vi "运维调试_总磷总氮.vi"() -> ()   [LabVIEW 2016, in "斯坦道仪器.lvlib"]
uses:
  <vilib>/Platform/TimedLoop/XDataNode/timing_clust.ctl
  <vilib>/Platform/TimedLoop/XDataNode/nitl_modes.ctl
  <vilib>/Platform/TimedLoop/XDataNode/wakeup.ctl
  <vilib>/Utility/miscctls.llb/LVPointTypeDef.ctl
  <vilib>/Utility/config.llb/Read Key (Double).vi
  <vilib>/Utility/config.llb/Write Key (Double).vi
  <vilib>/Platform/TimedLoop/XDataNode/XDataNode.xnode
  <vilib>/Platform/TimedLoop/XDataNode/XDNodeRunTimeDep.lvlib
  <vilib>/Utility/config.llb/NI_LVConfig.lvlib
panel:
  out "温度2":sgl
  out "温度1":sgl
  out "ADC":sgl
  out "字符串":string
  out "总氮稀释倍数":dbl
  out "固件版本号":string
  in  "数组":string[](array[string])
  in  "备用系数写入":bool
  in  "备用系数读取":bool
  in  "备用系数":T1
  in  "量程切换阈值写入":bool
  in  "量程切换阈值读取":bool
  in  "量程切换阈值":cluster{"阈值":dbl, "标液浓度":dbl}
  in  "参数下拉列表":enum16{"总磷", "总氮"}(ring)
  in  "量程下拉列表":enum16{"低量程", "高量程"}(ring)
  in  "测量模式下拉列表":enum16{"水样测量", "空白核查", "跨度核查", "标样核查", "加标回收"}(ring)
  in  "公式":cluster{"X^2":dbl, "X":dbl, "b":dbl}
  in  "写公式":bool
  in  "读公式":bool
  in  "精度":dbl=4.0
  in  "样品5 F0":dbl
  in  "样品5 F1":dbl
  in  "样品4 F1":dbl
  in  "样品4 F0":dbl
  in  "样品3 F0":dbl
  in  "样品3 F1":dbl
  in  "样品2 F0":dbl
  in  "样品2 F1":dbl
  in  "样品1 F1":dbl
  in  "样品1 F0":dbl
  in  "method":u16(ring) items=["最小二乘", "最小绝对残差", "Bisquare"]
  in  "模型":enum32{"线性", "多项式"}(ring)
  out "r^2":dbl format="%.7g"
  out "拟合公式":string
  in  "样品2启用":bool
  in  "样品5启用":bool
  in  "样品4启用":bool
  in  "样品3启用":bool
  in  "样品1启用":bool
  in  "标液浓度5":dbl
  out "测量吸光度5":dbl
  in  "标液浓度4":dbl
  out "测量吸光度4":dbl
  in  "标液浓度3":dbl
  out "测量吸光度3":dbl
  in  "标液浓度2":dbl
  out "测量吸光度2":dbl
  out "测量吸光度1":dbl
  in  "标液浓度1":dbl
  out "XY图":cluster{"X Values":dbl[], "Y Values":dbl[]}[](graph)
  in  "返回":bool
  in  "设置":bool
  out "序列号":string="序列号"
  out "总氮测量数据":T2(xcontrol)
  out "总磷测量数据":T2(xcontrol)
  out "集成报警信息":string
  out "设置值":dbl
  out "定时启动":bool
  out "总磷总氮运行状态":T3(xcontrol)
  in  "停止":bool
  in  "手动启动":bool
  in  "单步测试":bool
  in  "总磷氨氮调试":u16[](xcontrol)
  out "F3":sgl format="%#.6f"
  out "F2":sgl format="%#.6f"
  out "F1":sgl format="%#.6f"
  out "F0":sgl format="%#.6f"
  out "多列列表框":i32(listbox)
  # "COM5"
  # "参数设置"
  # "标液浓度"
  # "F0"
  # "F1"
  # "吸光值显示"
  # "样品一"
  # "辅\n助\n计\n算\n区"
  # "样品二"
  # "样品三"
  # "样品四"
  # "样品五"
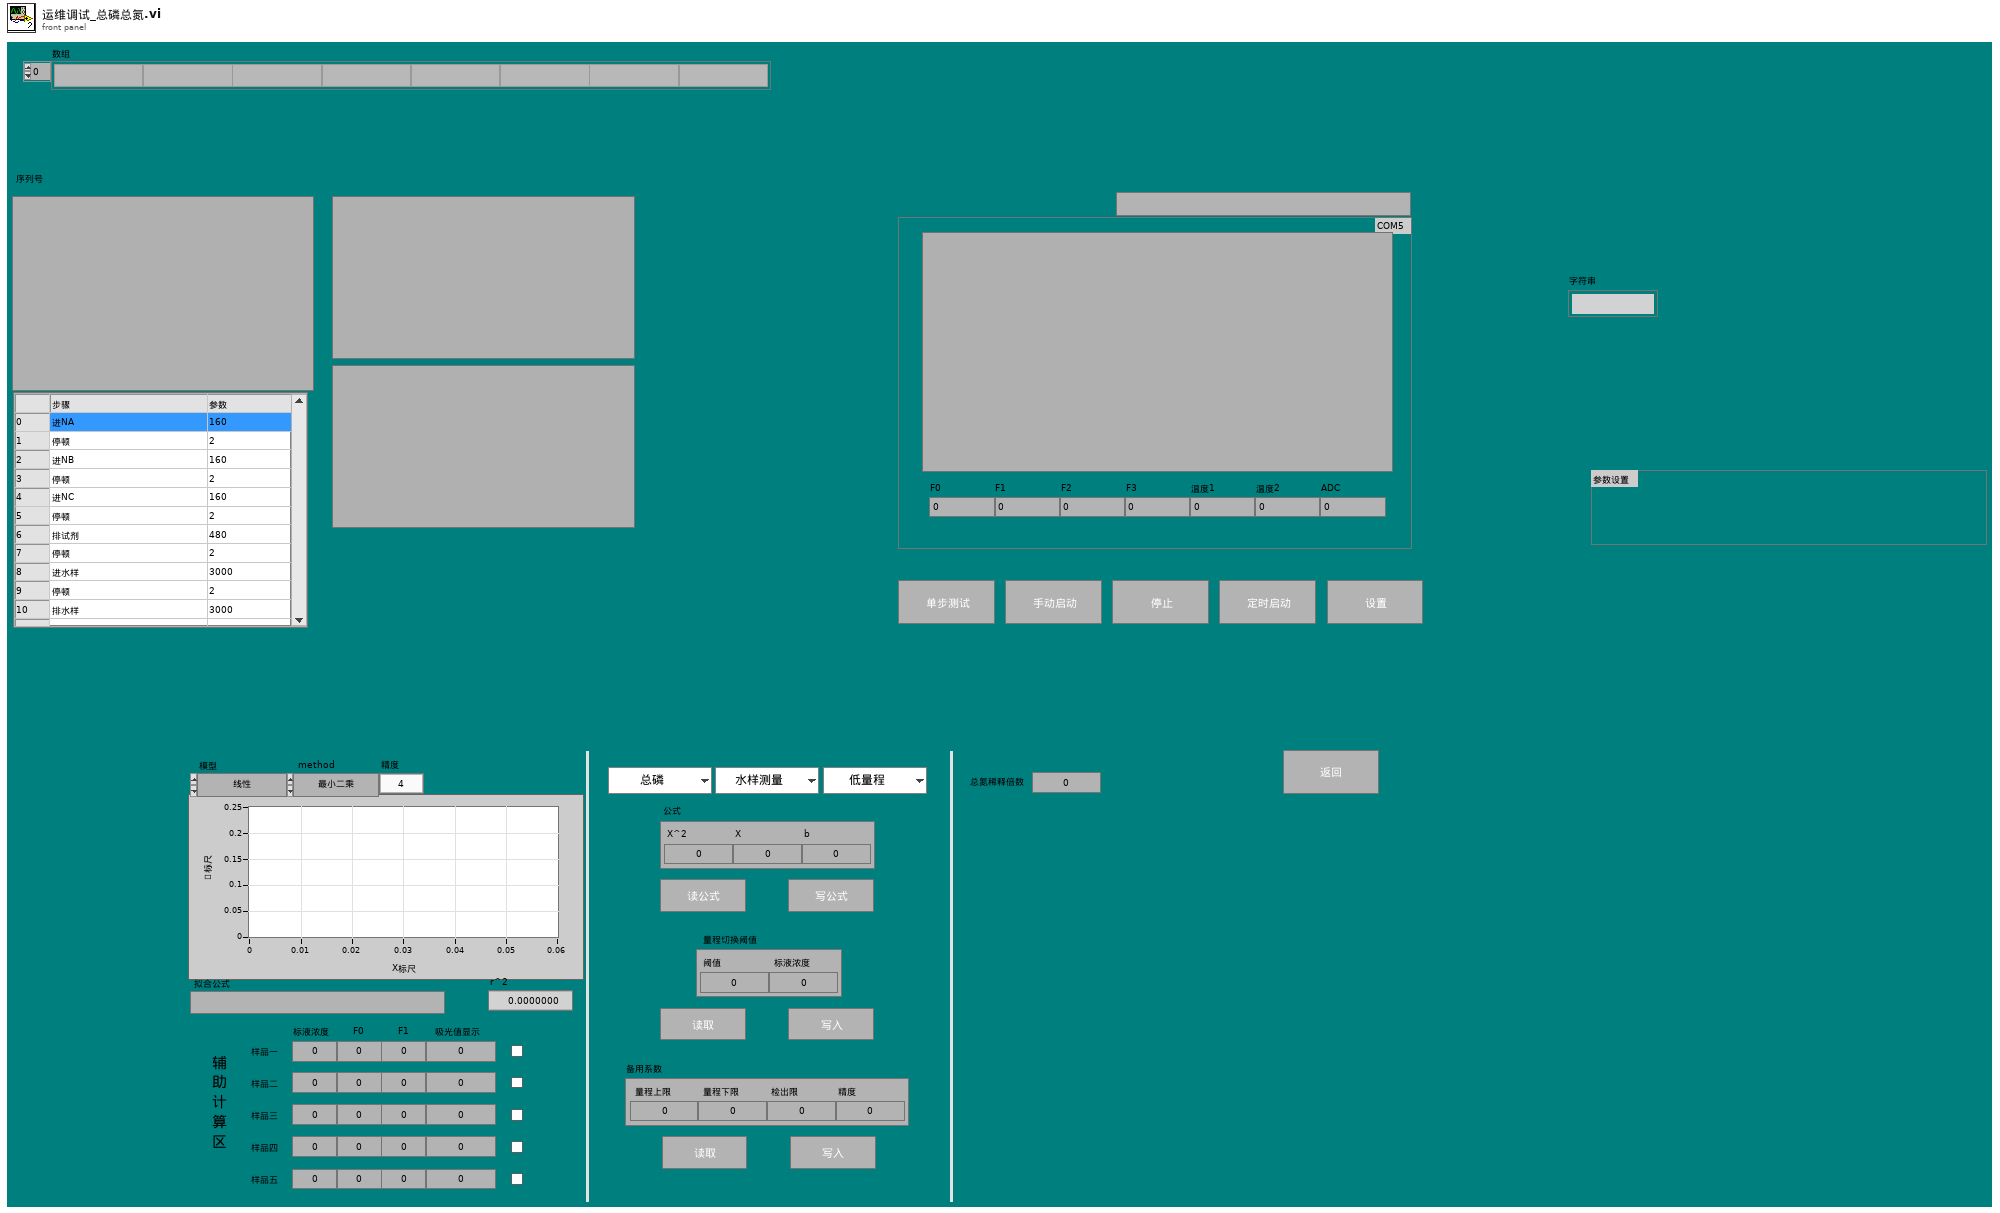
[diagram p1: front panel]
types:
  T1 = cluster{"量程上限":dbl, "量程下限":dbl, "检出限":dbl, "精度":dbl}
  T2 = cluster{"flowid":u16, "测量精度":u16, "测量数据区":cluster{"因子编码":u32, "单位":u16, "标样参考值":sgl, "水样数据时间":timestamp, "水样实测值":sgl, "水样数据标识":string, "标样数据时间":timestamp, "标样实测值":sgl, "标样数据标识":string, "空白数据时间":timestamp, "空白实测值":sgl, "空白数据标识":string, "零点核查数据时间":timestamp, "零点核查实测值":sgl, "零点核查数据标识":string, "跨度核查数据时间":timestamp, "跨度核查实测值":sgl, "跨度核查数据标识":string, "加标回收数据时间":timestamp, "加标回收实测值":sgl, "加标回收数据标识":string, "平行样数据时间":timestamp, "平行样实测值":sgl, "平行样数据标识":string, "F0":sgl, "F1":sgl, "F2":sgl, "F3":sgl, "F4":sgl, "F5":sgl, "F6":sgl, "F7":sgl, "温度":sgl, "湿度":sgl, "X值":sgl}}
  T3 = cluster{"系统时间":timestamp, "工作状态":enum16{"空闲", "水样测试", "标样核查", "零点核查", "跨度核查", "空白测试", "平行样测试", "加标回收", "空白校准", "标样校准", "初始化（清洗）"}, "测量模式":enum16{"待机", "连续模式", "周期模式", "定点模式", "受控模式", "手动模式"}, "告警代码":enum16{"无告警", "缺试剂告警", "缺水样告警", "缺蒸馏水告警", "缺标液告警", "仪表漏液告警", "标定异常告警", "超量程告警", "加热异常", "低试剂预警", "超上限告警", "超下限告警", "仪表内部其他异常", "滴定异常告警", "电极异常告警", "量程切换告警", "参数设置告警", "PH电极电位异常", "电导率电极异常", "浊度光度异常", "溶解氧电极异常", "溶解氧光强异常", "温度异常告警", "PH异常告警", "溶解氧异常告警", "电导率异常告警", "浊度异常告警", "叶绿素异常告警", "藻密度异常告警", "蓝绿藻异常告警", "ORP异常告警", "氨氮异常告警", "清洁刷异常告警", "SD卡异常告警", "蓝牙异常告警", "Wifi异常告警", "流程异常告警"}, "故障代码":enum16{"无故障", "电机故障", "温度故障", "通讯故障", "滴定故障"}, "日志代码":u16, "软件版本":u16, "F0":sgl, "F1":sgl, "F2":sgl, "F3":sgl, "T":sgl, "H":sgl, "id":u16, "flowid":u16, "量程":u16, "总磷控温温度1":sgl, "营养盐控温温度2":sgl, "ADC":sgl}
  T4 = enum16{"待机", "启动氨氮", "氨氮测量中", "启动总磷", "总磷测量中", "延时"}
  T5 = typedef "LVPointTypeDef.ctl" = cluster{"Horizontal":i16, "Vertical":i16}
  T6 = cluster{"因子编码":u32, "单位":u16, "标样参考值":sgl, "水样数据时间":timestamp, "水样实测值":sgl, "水样数据标识":string, "标样数据时间":timestamp, "标样实测值":sgl, "标样数据标识":string, "空白数据时间":timestamp, "空白实测值":sgl, "空白数据标识":string, "零点核查数据时间":timestamp, "零点核查实测值":sgl, "零点核查数据标识":string, "跨度核查数据时间":timestamp, "跨度核查实测值":sgl, "跨度核查数据标识":string, "加标回收数据时间":timestamp, "加标回收实测值":sgl, "加标回收数据标识":string, "平行样数据时间":timestamp, "平行样实测值":sgl, "平行样数据标识":string, "F0":sgl, "F1":sgl, "F2":sgl, "F3":sgl, "F4":sgl, "F5":sgl, "F6":sgl, "F7":sgl, "温度":sgl, "湿度":sgl, "X值":sgl}
  T7 = enum16{"空闲", "水样测试", "标样核查", "零点核查", "跨度核查", "空白测试", "平行样测试", "加标回收", "空白校准", "标样校准", "初始化（清洗）"}
  T8 = typedef "XDNodeRunTimeDep.lvlib/timing_clust.ctl" = cluster{"Expected End [f-1]":u64, "Actual End [f-1]":u64, "Finished Late? [f-1]":bool, "Expected End [i-1]":u64, "Actual End [i-1]":u64, "Finished Late? [i-1]":bool, "Expected Start [i]":u64, "Actual Start [i]":u64, "Expected Start [f]":u64, "Actual Start [f]":u64, "Source Name":string, "Structure Name":string, "Period":i64, "Deadline":i64, "Offset":i64, "Start":i64, "Priority":i32, "Timeout":i32, "Mode":T9, "Wakeup Reason":T10, "Error":errorcluster, "Source Type":string, "Secondary Source Type":string, "Global End Time":u64, "Global Start Time":u64, "Frame Duration":u64, "Iteration Duration":u64, "Assigned CPU":i32, "I/O Scan Engine Mode":u32}
  T9 = typedef "XDNodeRunTimeDep.lvlib/nitl_modes.ctl" = enum32{"No Change", "Process missed periods, maintain original phase", "Discard missed periods, maintain original phase", "Process missed periods, ignore original phase", "Discard missed periods, ignore original phase"}
  T10 = typedef "XDNodeRunTimeDep.lvlib/wakeup.ctl" = enum32{"Normal", "Aborted", "Asynchronous wakeup", "Timing source error", "Timed loop error", "Timeout"}
  T11 = cluster{"启动模式":enum16{"标液测量", "水样测量", "零液测量", "盲样测量", "加标回收"}, "启动参数":u16, "量程":enum16{"低量程", "高量程"}}
  T12 = cluster{"时间标识":timestamp, "设备":string, "日志信息":string, "流程参数":string}
  T13 = cluster{"时间标识":timestamp, "设备":string, "日志信息":string}
  T14 = enum16{"无告警", "缺试剂告警", "缺水样告警", "缺蒸馏水告警", "缺标液告警", "仪表漏液告警", "标定异常告警", "超量程告警", "加热异常", "低试剂预警", "超上限告警", "超下限告警", "仪表内部其他异常", "滴定异常告警", "电极异常告警", "量程切换告警", "参数设置告警", "PH电极电位异常", "电导率电极异常", "浊度光度异常", "溶解氧电极异常", "溶解氧光强异常", "温度异常告警", "PH异常告警", "溶解氧异常告警", "电导率异常告警", "浊度异常告警", "叶绿素异常告警", "藻密度异常告警", "蓝绿藻异常告警", "ORP异常告警", "氨氮异常告警", "清洁刷异常告警", "SD卡异常告警", "蓝牙异常告警", "Wifi异常告警", "流程异常告警"}
  T15 = typedef "LVRowAndColumnUnsignedTypeDef.ctl" = cluster{"Row":u32, "Column":u32}
  T16 = typedef "NI_LVConfig.lvlib/Config Data RefNum.ctl" = refnum<k1>
  T17 = cluster{"站号":u16, "量程切换":enum32{"H", "L", "AUTO"}, "控制命令":enum16{"启动测量", "标样核查", "零点核查", "跨度核查", "空白测试", "平行样测试", "加标回收", "空白校准", "标样校准", "初始化（清洗）", "停止测试", "仪器重启", "校时", "模式设置", "测量间隔设置"}, "模式设置":enum16{"待机", "连续模式", "周期模式", "定点模式", "受控模式", "手动模式"}, "测量间隔":u16}
  T18 = cluster{"站号":u16, "量程切换":enum32{"H", "L", "AUTO"}, "控制命令":enum16{"启动测量", "标样核查", "零点核查", "跨度核查", "空白测试", "平行样测试", "加标回收", "空白校准", "标样校准", "初始化（清洗）", "停止测试", "仪器重启", "校时", "模式设置", "测量间隔设置", "盲样测试"}, "模式设置":enum16{"待机", "连续模式", "周期模式", "定点模式", "受控模式", "手动模式"}, "测量间隔":u16}
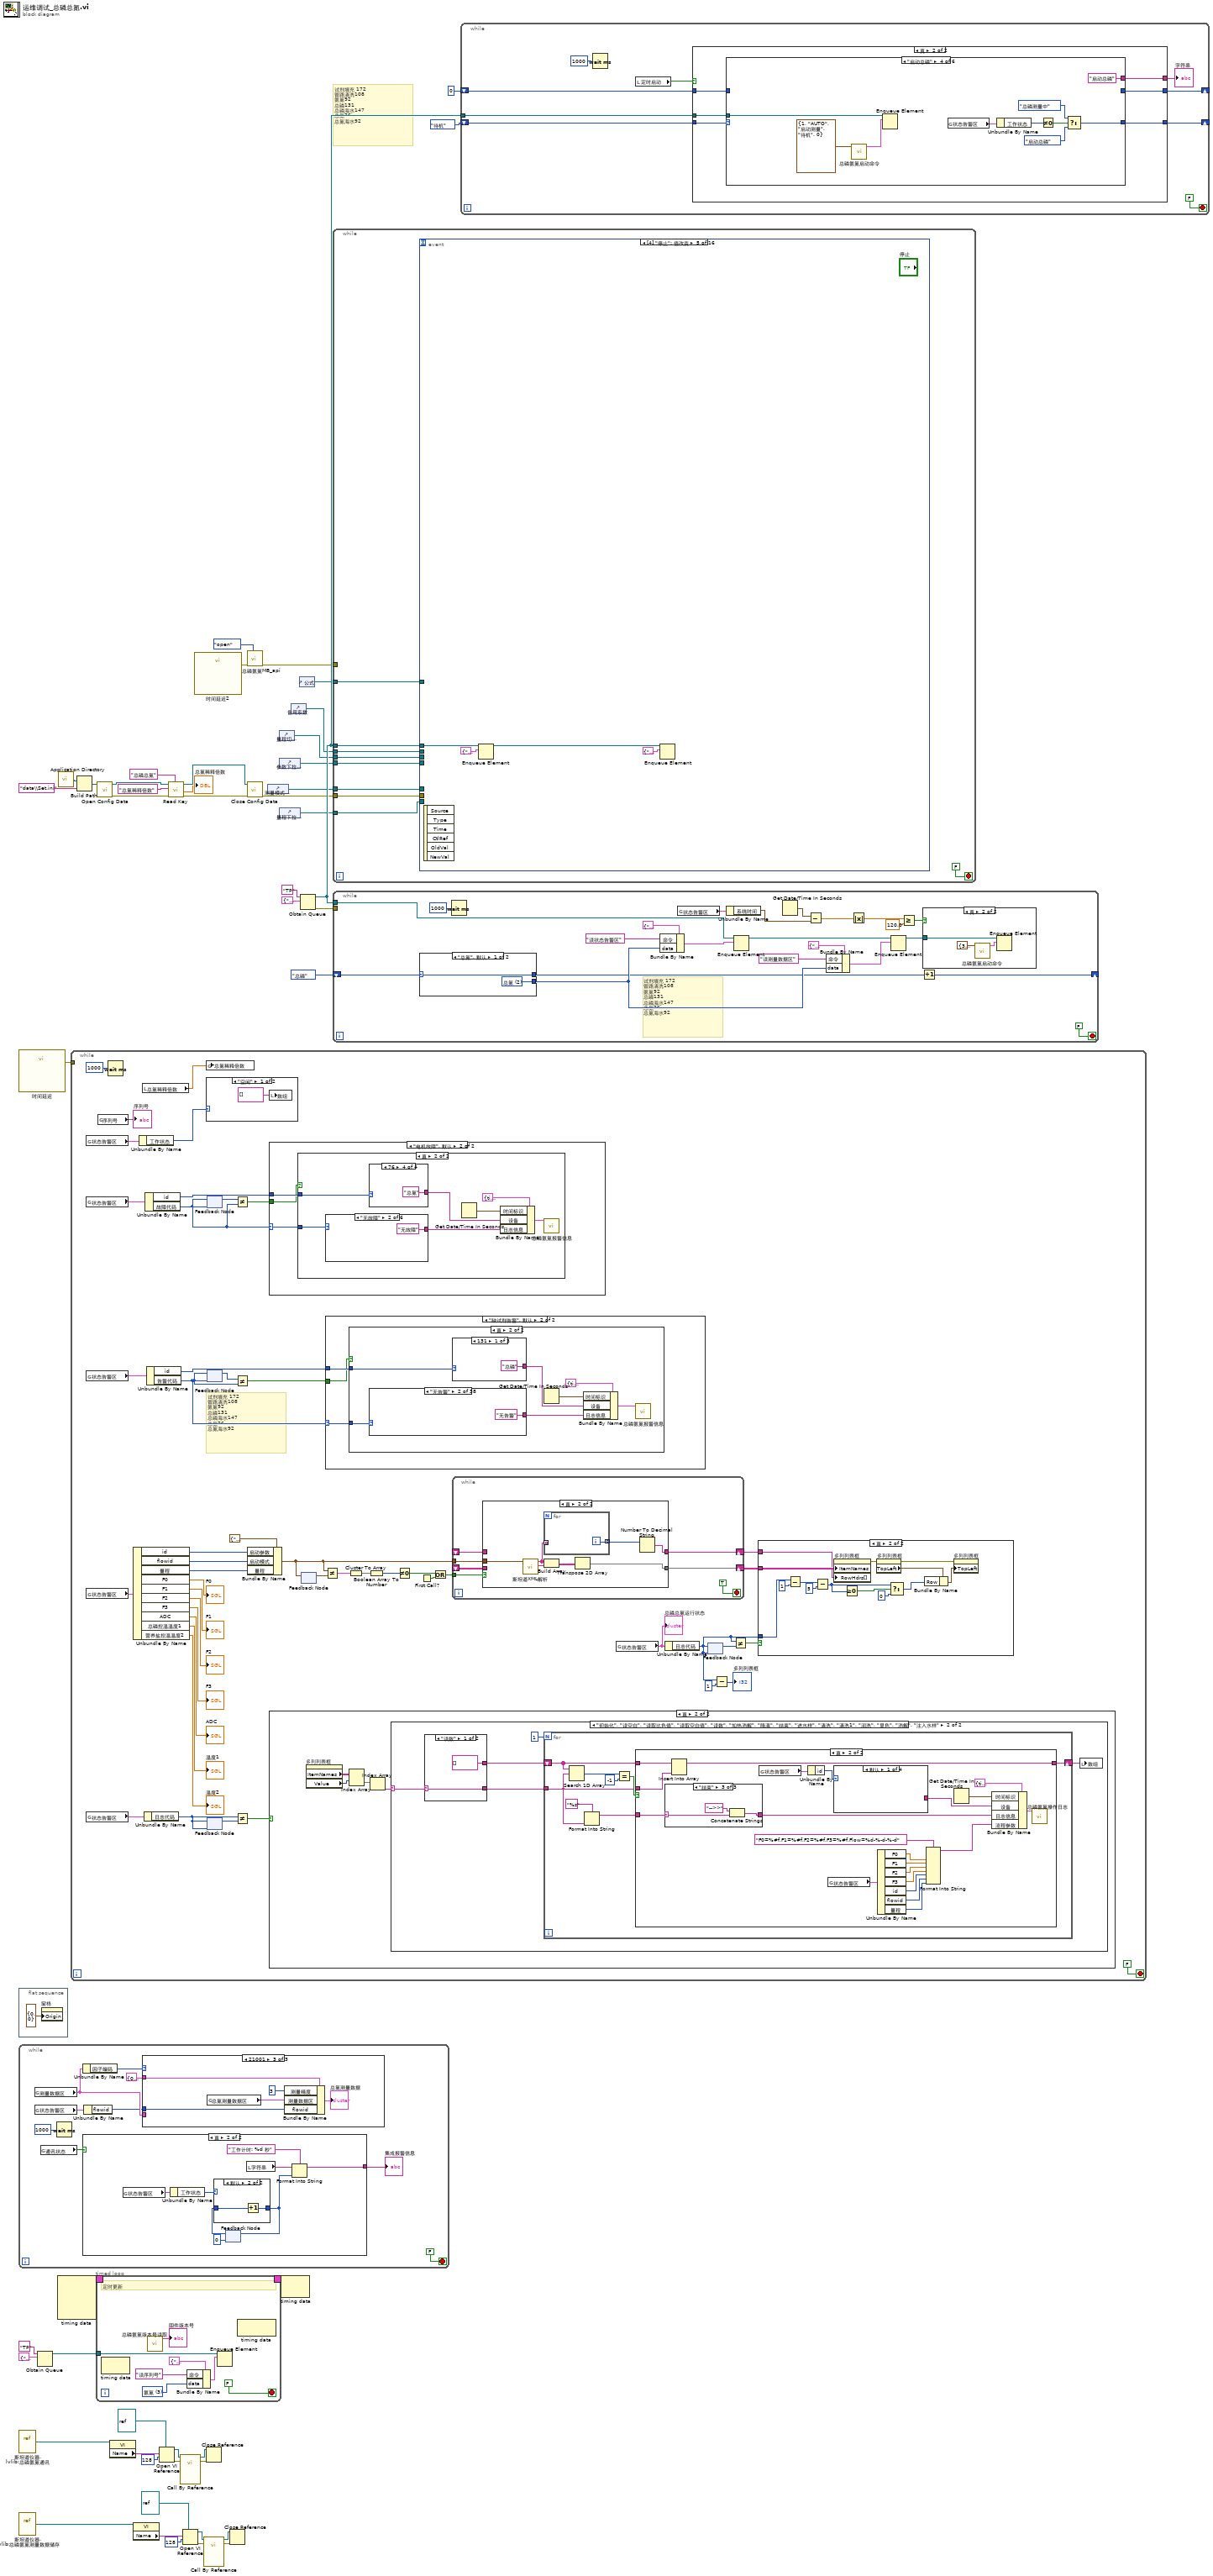
[diagram p0: block diagram]
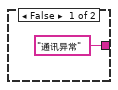
[diagram p2: hidden frame]
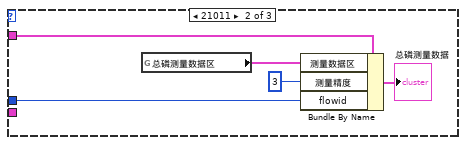
[diagram p5: hidden frame]
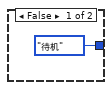
[diagram p6: hidden frame]
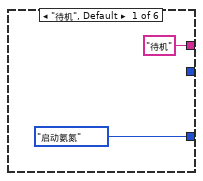
[diagram p7: hidden frame]
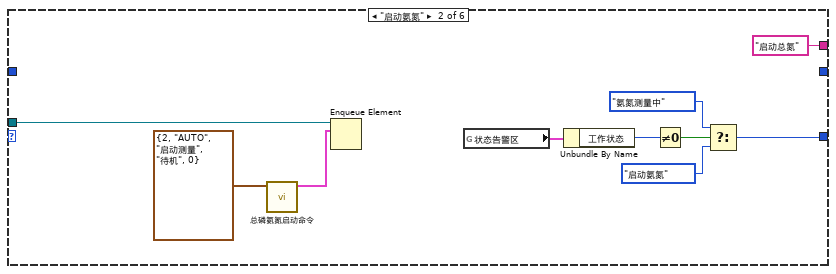
[diagram p8: hidden frame]
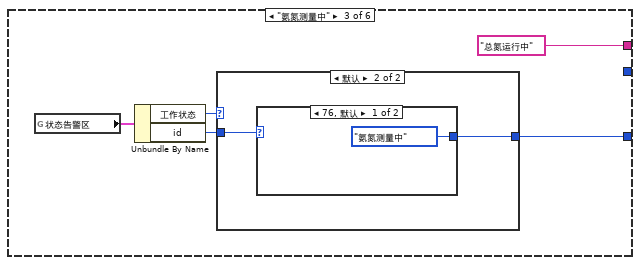
[diagram p9: hidden frame]
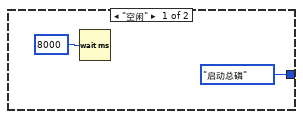
[diagram p10: hidden frame]
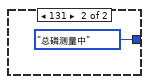
[diagram p11: hidden frame]
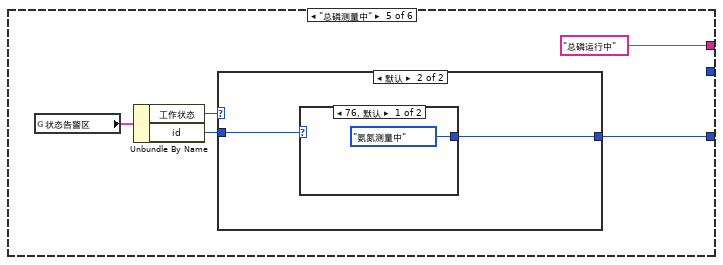
[diagram p12: hidden frame]
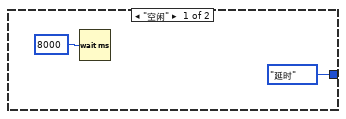
[diagram p13: hidden frame]
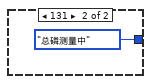
[diagram p14: hidden frame]
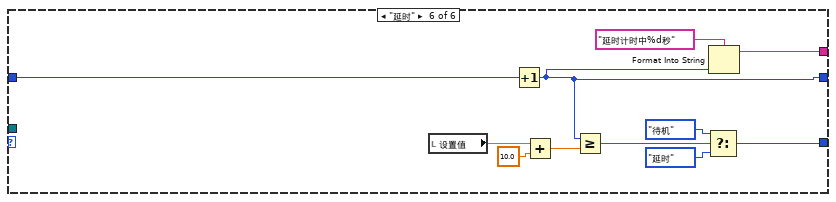
[diagram p15: hidden frame]
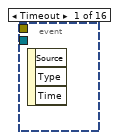
[diagram p16: hidden frame]
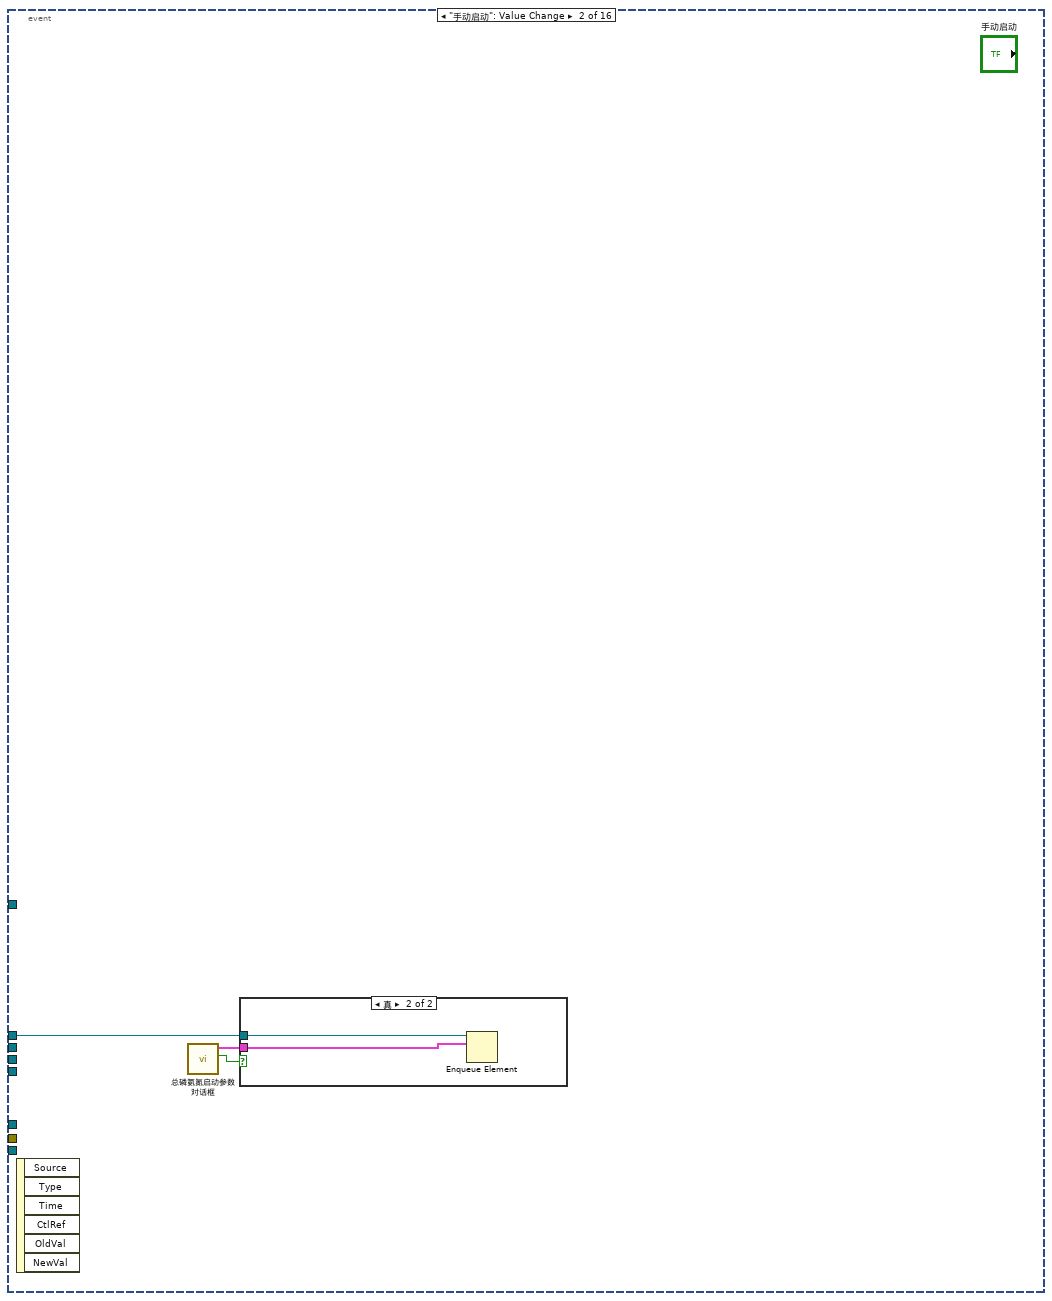
[diagram p17: hidden frame]
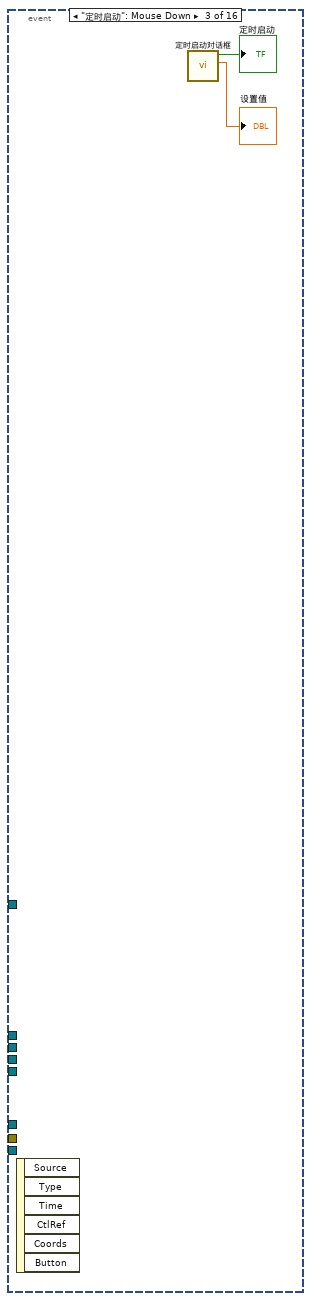
[diagram p19: hidden frame]
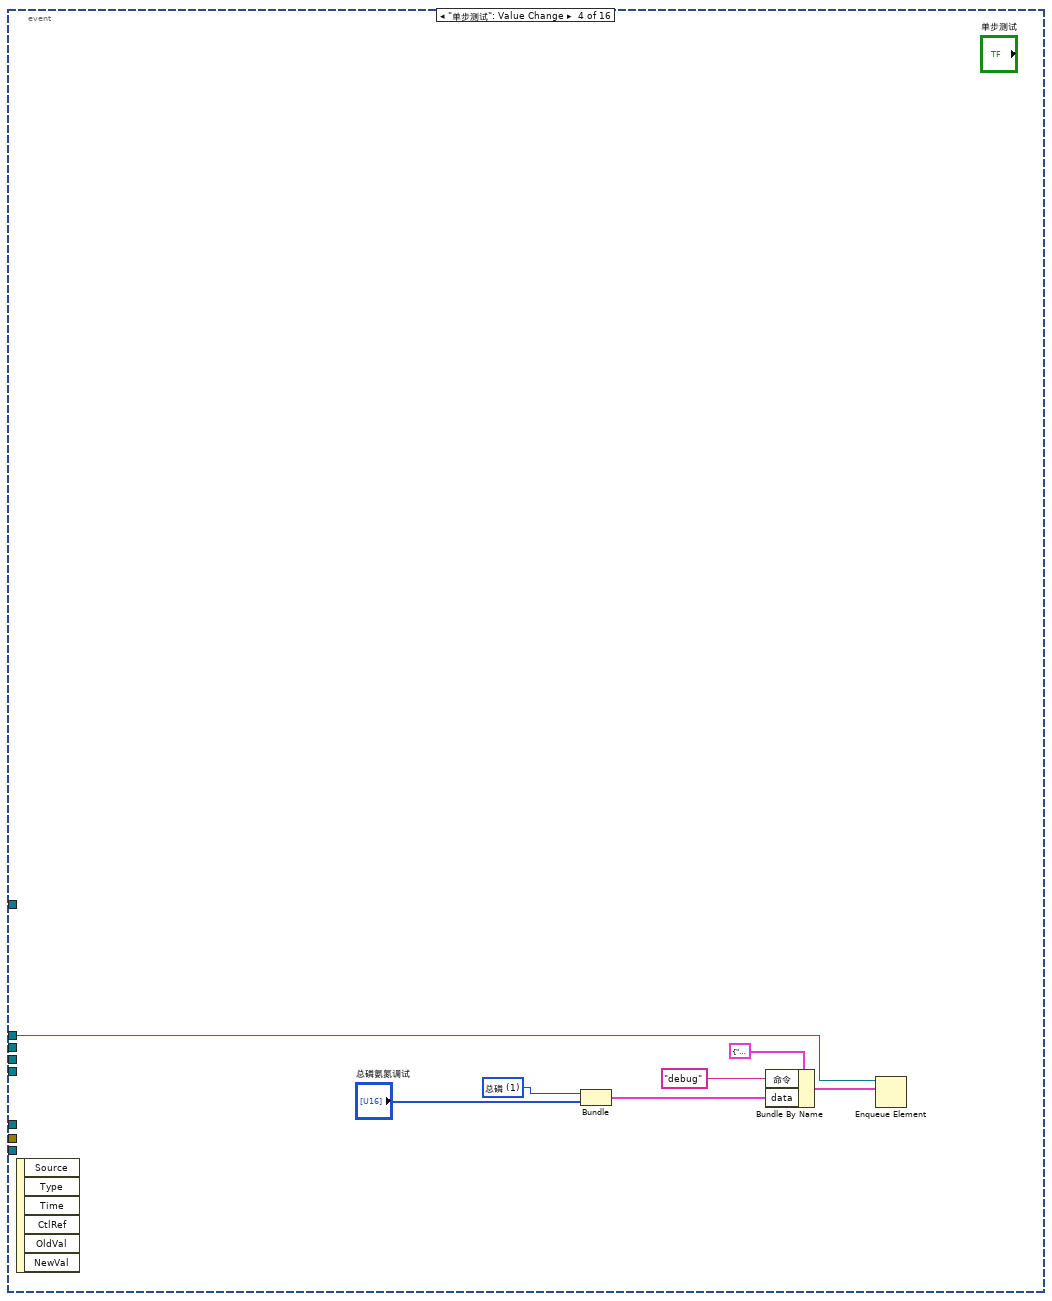
[diagram p20: hidden frame]
diagram:
  # "试剂填充 172 \n管路清洗108\n氨氮92\n总磷131\n总磷海水147\n总氮76\n总氮海水92"
  n1 = call "时间延迟"() -> ("error out"=w20:errorcluster)  [unwired: 11 in]
  n2 = flat-sequence {
    frame #0 {
      n3 = property on="窗格" class="Pane"("Origin"=T5 {"Horizontal"=0, "Vertical"=0} ("原点")) -> ()  [unwired: 2 in, 2 out]
    }
  }
  n4 = while {
    stop <- FALSE stop-if-true
    n5 = global read "VAR总磷氨氮全局变量.vi" "测量数据区"() -> (w57:T6)
    n6 = global read "VAR总磷氨氮全局变量.vi" "状态告警区"() -> (w53:T3)
    n7 = global read "VAR总磷氨氮全局变量.vi" "通讯状态"() -> (w55:bool)
    n8 = Wait (ms)(milliseconds to wait=u32 1000 ("等待时间（毫秒）")) -> ()  [unwired: 1 out]
    n9 = Unbundle By Name(w57) -> ("因子编码"=w56:u32)
    n10 = case shown="真" w55 {
      tunnel: ["通讯异常" ("集成报警信息") w62] -> w54
      frame False {
      }
      frame True {
        n11 = global read "VAR总磷氨氮全局变量.vi" "状态告警区"() -> (w68:T3)
        n12 = Unbundle By Name(w68) -> ("工作状态"=w67:T7)
        n13 = feedback #1(0) -> (w65:i32)
        n14 = case shown="默认" w67 {
          tunnel: w65 -> [_ w70]
          tunnel: [_ w69] -> w63
          frame "空闲" {
          }
          frame Default {
            n15 = Increment(x=w70) -> (x+1=w69:i32)
          }
        }
        n16 = feedback-in #1(w63) -> ()
        n17 = local read "字符串"() -> (w61:string)
        n18 = Format Into String(format string="工作计时: %d 秒" ("格式字符串"), initial string=w61, w63) -> (resulting string=w62:string)  [unwired: 1 in, 1 out]
      }
    }
    "集成报警信息" <- w54
    n19 = Unbundle By Name(w53) -> ("flowid"=w52:u16)
    n20 = case shown="21001" w56 {
      tunnel: w57 -> [_ _ _]
      tunnel: w52 -> [_ w73 w79]
      tunnel: T2 {"flowid"=0, "测量精度"=0, "测量数据区"={"因子编码"=0, "单位"=0, "标样参考值"=0.0, "水样数据时间"=timestamp(0 s since 1904-01-01), "水样实测值"=0.0, "水样数据标识"="", "标样数据时间"=timestamp(0 s since 1904-01-01), "标样实测值"=0.0, "标样数据标识"="", "空白数据时间"=timestamp(0 s since 1904-01-01), "空白实测值"=0.0, "空白数据标识"="", "零点核查数据时间"=timestamp(0 s since 1904-01-01), "零点核查实测值"=0.0, "零点核查数据标识"="", "跨度核查数据时间"=timestamp(0 s since 1904-01-01), "跨度核查实测值"=0.0, "跨度核查数据标识"="", "加标回收数据时间"=timestamp(0 s since 1904-01-01), "加标回收实测值"=0.0, "加标回收数据标识"="", "平行样数据时间"=timestamp(0 s since 1904-01-01), "平行样实测值"=0.0, "平行样数据标识"="", "F0"=0.0, "F1"=0.0, "F2"=0.0, "F3"=0.0, "F4"=0.0, "F5"=0.0, "F6"=0.0, "F7"=0.0, "温度"=0.0, "湿度"=0.0, "X值"=0.0}} ("总氮测量数据") -> [_ w72 w78]
      frame Default {
      }
      frame 21011 {
        n21 = global read "VAR总磷氨氮全局变量.vi" "总磷测量数据区"() -> (w71:T6)
        n22 = Bundle By Name(cluster=w72, "测量数据区"=w71, "测量精度"=u16 3, "flowid"=w73) -> (→"总磷测量数据":T2)
      }
      frame 21001 {
        n23 = global read "VAR总磷氨氮全局变量.vi" "总氮测量数据区"() -> (w76:T6)
        n24 = Bundle By Name(cluster=w78, "测量精度"=u16 3, "测量数据区"=w76, "flowid"=w79) -> (→"总氮测量数据":T2)
      }
    }
  }
  n25 = vi-ref "斯坦道仪器.lvlib:总磷氨氮通讯.vi"() -> (w43:refnum<vi>)
  n26 = vi-ref "斯坦道仪器.lvlib:总磷氨氮测量数据储存.vi"() -> (w35:refnum<vi>)
  n27 = Obtain Queue(name (unnamed)="TP" ("名称（未命名）"), element data type=cluster{"命令":string, "data":variant} {"命令"="", "data"=variant}) -> (queue out=w13:refnum<queue>)  [unwired: 3 in, 2 out]
  n28 = node-c288() -> (w17:T8)  [unwired: 4 in]
  n29 = call <vilib>:"Application Directory.vi"() -> ("Application Directory"=w7:path)
  n30 = while {
    tunnel: w20 -> [_]
    stop <- FALSE stop-if-true
    # "试剂填充 172 \n管路清洗108\n氨氮92\n总磷131\n总磷海水147\n总氮76\n总氮海水92"
    n31 = global read "VAR总磷氨氮全局变量.vi" "状态告警区"() -> (w93:T3)
    n32 = global read "VAR总磷氨氮全局变量.vi" "状态告警区"() -> (w98:T3)
    n33 = global read "VAR总磷氨氮全局变量.vi" "状态告警区"() -> (w103:T3)
    n34 = global read "VAR总磷氨氮全局变量.vi" "状态告警区"() -> (w115:T3)
    n35 = global read "VAR总磷氨氮全局变量.vi" "状态告警区"() -> (w90:T3)
    n36 = global read "VAR总磷氨氮全局变量.vi" "序列号"() -> (→"序列号":string)
    n37 = Wait (ms)(milliseconds to wait=u32 1000 ("等待时间（毫秒）")) -> ()  [unwired: 1 out]
    n38 = Unbundle By Name(w115) -> ("id"=w112:u16, "flowid"=w114:u16, "量程"=w113:u16, "F0"=→"F0":sgl, "F1"=→"F1":sgl, "F2"=→"F2":sgl, "F3"=→"F3":sgl, "ADC"=→"ADC":sgl, "总磷控温温度1"=→"温度1":sgl, "营养盐控温温度2"=→"温度2":sgl)
    n39 = Unbundle By Name(w93) -> ("工作状态"=w92:T7)
    n40 = local read "总氮稀释倍数"() -> (w84:dbl)
    n41 = Unbundle By Name(w90) -> ("日志代码"=w89:u16)
    n42 = Unbundle By Name(w98) -> ("id"=w97:u16, "故障代码"=w94:enum16{"无故障", "电机故障", "温度故障", "通讯故障", "滴定故障"})
    n43 = Unbundle By Name(w103) -> ("id"=w102:u16, "告警代码"=w99:T14)
    n44 = global write "VAR总磷氨氮全局变量.vi" "总氮稀释倍数"(w84) -> ()
    n45 = case shown="\"空闲\"" w92 {
      frame "空闲" {
        n46 = local write "数组"(string[] [] ("数组")) -> ()
      }
      frame "水样测试", Default {
      }
    }
    n47 = feedback #2(w94) -> (w95:enum16{"无故障", "电机故障", "温度故障", "通讯故障", "滴定故障"})
    n48 = feedback-in #2(w94) -> ()
    n49 = feedback #3(w99) -> (w100:T14)
    n50 = feedback-in #3(w99) -> ()
    n51 = feedback #4(w89) -> (w91:u16)
    n52 = feedback-in #4(w89) -> ()
    n53 = Not Equal?(x=w95, y=w94) -> (x != y?=w96:bool)
    n54 = Not Equal?(x=w100, y=w99) -> (x != y?=w101:bool)
    n55 = Not Equal?(x=w89, y=w91) -> (x != y?=w88:bool)
    n56 = Bundle By Name(cluster=T11 {"启动模式"=enum."加标回收", "启动参数"=1, "量程"=enum."低量程"} ("参数簇"), "启动参数"=w112, "启动模式"=w114, "量程"=w113) -> (w105:T11)
    n57 = case shown="\"电机故障\", 默认" w94 {
      selector: w94 -> [_ w184]
      tunnel: w97 -> [_ w185]
      tunnel: w96 -> [_ w183]
      frame "无故障" {
      }
      frame "电机故障", Default {
        n58 = case shown="真" w183 {
          tunnel: w185 -> [_ w192]
          tunnel: w184 -> [_ w187]
          frame False {
          }
          frame True {
            n59 = case shown="\"无故障\"" w187 {
              selector: w187 -> [w194 _ _ _ _ _]
              tunnel: [w193 "无故障" "电机故障" "温度故障" "通讯故障" "滴定故障"] -> w186
              frame Default {
                n60 = Format Into String(format string="%d" ("格式字符串"), initial string="未知" ("工作状态"), w194) -> (resulting string=w193:string)  [unwired: 1 in, 1 out]
              }
              frame "无故障" {
              }
              frame "电机故障" {
              }
              frame "温度故障" {
              }
              frame "通讯故障" {
              }
              frame "滴定故障" {
              }
            }
            n61 = case shown="76" w192 {
              tunnel: [_ "总磷" ("table输入") "氨氮" ("table输入") "总氮" ("table输入")] -> w188
              frame Default {
              }
              frame 131 {
              }
              frame 92 {
              }
              frame 76 {
              }
            }
            n62 = Get Date/Time In Seconds() -> (seconds since 1Jan1904=w189:timestamp)
            n63 = Bundle By Name(cluster=T13 {"时间标识"=timestamp(0 s since 1904-01-01), "设备"="", "日志信息"=""} ("data in"), "时间标识"=w189, "设备"=w188, "日志信息"=w186) -> (w190:T13)
            n64 = call "总磷氨氮报警信息.vi"("data in"=w190) -> ()  [unwired: 11 in]
          }
        }
      }
    }
    n65 = case shown="真" w88 {
      frame False {
      }
      frame True {
        n66 = property on="多列列表框" class="MCListbox (严格)"() -> ("ItemNames"=w132:string[][], "Value"=w133:i32)  [unwired: 2 in, 2 out]
        n67 = Index Array(array=w132, index (row)=w133) -> (element=w131:string[])  [unwired: 1 in]
        n68 = Index Array(array=w131) -> (element=w130:string)  [unwired: 1 in]
        n69 = case shown="\"初始化\", \"读空白\", \"读取比色值\", \"读取空白值\", \"读数\", \"加热消解\", \"降温\", \"结束\", \"进水样\", \"清洗\", \"清洗1\", \"润洗\", \"显色\", \"消解\", \"注入水样\"" w130 {
          selector: w130 -> [_ w136]
          frame Default {
          }
          frame "初始化", "读空白", "读取比色值", "读取空白值", "读数", "加热消解", "降温", "结束", "进水样", "清洗", "清洗1", "润洗", "显色", "消解", "注入水样" {
            n70 = case shown="\"读数\"" w136 {
              selector: w136 -> [w140 w142]
              tunnel: [w140 w142] -> w135
              tunnel: [string[] [] ("数组") "数组"] -> w134
              frame "读数" {
              }
              frame Default {
              }
            }
            n71 = for {
              N: 1 -> [_]
              tunnel: w135 -> [w144]
              shift-right: [w143] -> w137
              shift-left: w134 -> [w145]
              n72 = Search 1D Array(1D array=w145, element=w144) -> (index of element=w148:i32)  [unwired: 1 in]
              n73 = Format Into String(format string="%s" ("格式字符串"), w144) -> (resulting string=w149:string)  [unwired: 2 in, 1 out]
              n74 = Equal?(x=w148, y=-1) -> (x = y?=w146:bool)
              n75 = case shown="真" w146 {
                tunnel: w149 -> [_ w153]
                tunnel: w145 -> [w151 w157]
                tunnel: w144 -> [_ w156]
                tunnel: [w151 w155] -> w143
                frame False {
                }
                frame True {
                  n76 = case shown="\"结束\"" w153 {
                    selector: w153 -> [w173 w176 w179]
                    tunnel: [w173 w175 w178] -> w152
                    frame Default {
                    }
                    frame "初始化" {
                      n77 = Concatenate Strings("-->>" ("字符串"), w176) -> (w175:string)
                    }
                    frame "结束" {
                      n78 = Concatenate Strings("-->>" ("字符串"), w179) -> (w178:string)
                    }
                  }
                  n79 = Insert Into Array(array=w157, new element=w156) -> (w155:string[])  [unwired: 1 in]
                  n80 = global read "VAR总磷氨氮全局变量.vi" "状态告警区"() -> (w172:T3)
                  n81 = Unbundle By Name(w172) -> ("id"=w171:u16)
                  n82 = global read "VAR总磷氨氮全局变量.vi" "状态告警区"() -> (w167:T3)
                  n83 = case shown="默认" w171 {
                    tunnel: [_ "总磷" ("table输入") "氨氮" ("table输入") "总氮" ("table输入")] -> w169
                    frame Default {
                    }
                    frame 131 {
                    }
                    frame 92 {
                    }
                    frame 76 {
                    }
                  }
                  n84 = Unbundle By Name(w167) -> ("F0"=w164:sgl, "F1"=w163:sgl, "F2"=w162:sgl, "F3"=w161:sgl, "id"=w160:u16, "flowid"=w159:u16, "量程"=w158:u16)
                  n85 = Format Into String(format string="F0=%#f,F1=%#f,F2=%#f,F3=%#f,Flow=%d-%-d-%-d" ("格式字符串"), w164, w163, w162, w161, w160, w159, w158) -> (resulting string=w165:string)  [unwired: 2 in, 1 out]
                  n86 = Get Date/Time In Seconds() -> (seconds since 1Jan1904=w168:timestamp)
                  n87 = Bundle By Name(cluster=T12 {"时间标识"=timestamp(0 s since 1904-01-01), "设备"="", "日志信息"="", "流程参数"=""} ("data in"), "时间标识"=w168, "设备"=w169, "日志信息"=w152, "流程参数"=w165) -> (w170:T12)
                  n88 = call "总磷氨氮操作日志.vi"("data in"=w170) -> ()  [unwired: 11 in]
                }
              }
            }
            n89 = local write "数组"(w137) -> ()
          }
        }
      }
    }
    n90 = feedback #5() -> (w121:T11)  [unwired: 1 in]
    n91 = feedback-in #5(w105) -> ()
    n92 = Not Equal?(x=w105, y=w121) -> (x != y?=w122:cluster{"启动模式":bool, "启动参数":bool, "量程":bool})
    n93 = case shown="\"缺试剂告警\", 默认" w99 {
      selector: w99 -> [_ w206]
      tunnel: w102 -> [_ w207]
      tunnel: w101 -> [_ w205]
      frame "无告警" {
      }
      frame "缺试剂告警", Default {
        n94 = case shown="真" w205 {
          tunnel: w207 -> [_ w214]
          tunnel: w206 -> [_ w208]
          frame False {
          }
          frame True {
            n95 = case shown="\"无告警\"" w208 {
              selector: w208 -> [w216 _ _ _ _ _ _ _ _ _ _ _ _ _ _ _ _ _ _ _ _ _ _ _ _ _ _ _ _ _ _ _ _ _ _ _ _ _]
              tunnel: [w215 "无告警" "缺试剂告警" "缺水样告警" "缺蒸馏水告警" "缺标液告警" "仪表漏液告警" "标定异常告警" "超量程告警" "加热异常" "低试剂预警" "超上限告警" "超下限告警" "仪表内部其他异常" "滴定异常告警" "电极异常告警" "量程切换告警" "参数设置告警" "PH电极电位异常" "电导率电极异常" "浊度光度异常" "溶解氧电极异常" "溶解氧光强异常" "温度异常告警" "PH异常告警" "溶解氧异常告警" "电导率异常告警" "浊度异常告警" "叶绿素异常告警" "藻密度异常告警" "蓝绿藻异常告警" "ORP异常告警" "氨氮异常告警" "清洁刷异常告警" "SD卡异常告警" "蓝牙异常告警" "WiFi异常告警" "流程异常告警"] -> w209
              frame Default {
                n96 = Format Into String(format string="%d" ("格式字符串"), initial string="未知" ("工作状态"), w216) -> (resulting string=w215:string)  [unwired: 1 in, 1 out]
              }
              frame "无告警" {
              }
              frame "缺试剂告警" {
              }
              frame "缺水样告警" {
              }
              frame "缺蒸馏水告警" {
              }
              frame "缺标液告警" {
              }
              frame "仪表漏液告警" {
              }
              frame "标定异常告警" {
              }
              frame "超量程告警" {
              }
              frame "加热异常" {
              }
              frame "低试剂预警" {
              }
              frame "超上限告警" {
              }
              frame "超下限告警" {
              }
              frame "仪表内部其他异常" {
              }
              frame "滴定异常告警" {
              }
              frame "电极异常告警" {
              }
              frame "量程切换告警" {
              }
              frame "参数设置告警" {
              }
              frame "PH电极电位异常" {
              }
              frame "电导率电极异常" {
              }
              frame "浊度光度异常" {
              }
              frame "溶解氧电极异常" {
              }
              frame "溶解氧光强异常" {
              }
              frame "温度异常告警" {
              }
              frame "PH异常告警" {
              }
              frame "溶解氧异常告警" {
              }
              frame "电导率异常告警" {
              }
              frame "浊度异常告警" {
              }
              frame "叶绿素异常告警" {
              }
              frame "藻密度异常告警" {
              }
              frame "蓝绿藻异常告警" {
              }
              frame "ORP异常告警" {
              }
              frame "氨氮异常告警" {
              }
              frame "清洁刷异常告警" {
              }
              frame "SD卡异常告警" {
              }
              frame "蓝牙异常告警" {
              }
              frame "Wifi异常告警" {
              }
              frame "流程异常告警" {
              }
            }
            n97 = case shown="131" w214 {
              tunnel: ["总磷" ("table输入") "氨氮" ("table输入") "总氮" ("table输入")] -> w210
              frame 131 {
              }
              frame 92 {
              }
              frame 76, Default {
              }
            }
            n98 = Get Date/Time In Seconds() -> (seconds since 1Jan1904=w211:timestamp)
            n99 = Bundle By Name(cluster=T13 {"时间标识"=timestamp(0 s since 1904-01-01), "设备"="", "日志信息"=""} ("data in"), "时间标识"=w211, "设备"=w210, "日志信息"=w209) -> (w212:T13)
            n100 = call "总磷氨氮报警信息.vi"("data in"=w212) -> ()  [unwired: 11 in]
          }
        }
      }
    }
    n101 = Cluster To Array(cluster=w122) -> (array=w123:bool[])
    n102 = Boolean Array To Number(Boolean array=w123) -> (number=w124:u32)
    n103 = Not Equal To 0?(x=w124) -> (x != 0?=w117:bool)
    n104 = First Call?() -> (First Call?: T/F=w118:bool)
    n105 = Or(x=w117, y=w118) -> (x .or. y?=w116:bool)
    n106 = while {
      tunnel: w116 -> [w265]
      tunnel: w105 -> [w264]
      shift-right: [w263] -> w120
      shift-left: _ -> [w259]
      shift-right: [w262] -> w119
      shift-left: _ -> [w260]
      stop <- TRUE stop-if-true
      n107 = case shown="真" w265 {
        tunnel: [w267 w274] -> w262
        tunnel: [w266 w273] -> w263
        tunnel: w264 -> [_ w268]
        tunnel: w260 -> [w267 _]
        tunnel: w259 -> [w266 _]
        frame False {
        }
        frame True {
          n108 = call "斯坦道XML解析.vi"("参数簇"=w268) -> ("步骤时间"=w269:string[], "步骤名"=w271:string[])  [unwired: 9 in]
          n109 = for {
            tunnel: w271 -> [_] mode=indexing
            tunnel: [w275] -> w272 mode=indexing
            i -> [w275]
          }
          n110 = Build Array(w271, w269) -> (w270:string[][])
          n111 = Transpose 2D Array(2D array=w270) -> (transposed array=w273:string[][])
          n112 = Number To Decimal String(number=w272) -> (decimal integer string=w274:string[])  [unwired: 1 in]
        }
      }
    }
    n113 = global read "VAR总磷氨氮全局变量.vi" "状态告警区"() -> (w106:T3)
    "总磷总氮运行状态" <- w106
    n114 = Unbundle By Name(w106) -> ("日志代码"=w86:u16)
    n115 = feedback-in #6(w86) -> ()
    n116 = feedback #6(w86) -> (w126:u16)
    n117 = Subtract(x=w86, y=1) -> (x-y=→"多列列表框":i32)
    n118 = Not Equal?(x=w86, y=w126) -> (x != y?=w125:bool)
    n119 = case shown="真" w125 {
      tunnel: w86 -> [_ w278]
      tunnel: w120 -> [_ w285]
      tunnel: w119 -> [_ w284]
      frame False {
      }
      frame True {
        n120 = Subtract(x=w278, y=1) -> (x-y=w276:i32)
        n121 = Subtract(x=w276, y=5) -> (x-y=w280:i32)
        n122 = property on="多列列表框" class="MCListbox (严格)"("ItemNames"=w285, "RowHdrs[]"=w284) -> (error out=w286:errorcluster)  [unwired: 2 in, 1 out]
        n123 = Greater Or Equal To 0?(x=w280) -> (x >= 0?=w279:bool)
        n124 = property on="多列列表框" class="MCListbox (严格)"(error in=w286) -> (error out=w287:errorcluster, "TopLeft"=w288:T15)  [unwired: 1 in, 1 out]
        n125 = Select(t=w280, s=w279, f=0) -> (s? t:f=w281:i32)
        n126 = Bundle By Name(cluster=w288, "Row"=w281) -> (w289:T15)
        n127 = property on="多列列表框" class="MCListbox (严格)"(error in=w287, "TopLeft"=w289) -> ()  [unwired: 1 in, 2 out]
      }
    }
  }
  n128 = Build Path(base path=w7, name or relative path="data\\Set.ini" ("名称或相对路径")) -> (appended path=w5:path)
  n129 = timed-loop {
    timing: w17 -> [_]
    timing-out: [_] -> w16
    tunnel: w13 -> [w292]
    stop <- FALSE stop-if-true
    w293 = u16 3 items=["总磷"=1, "氨氮"=3] ("站号")
    # "定时更新"
    n130 = node-c288() -> ()  [unwired: 1 in, 1 out]
    n131 = call "总磷氨氮版本号读取.vi"() -> ("固件版本号"=→"固件版本号":string)  [unwired: 11 in]
    n132 = Bundle By Name(cluster=cluster{"命令":string, "data":variant} {"命令"="", "data"=variant} ("元素"), "命令"="读序列号", "data"=w293) -> (w291:cluster{"命令":string, "data":variant})
    n133 = Enqueue Element(queue=w292, element=w291) -> ()  [unwired: 2 in, 3 out]
    n134 = node-c288() -> ()  [unwired: 1 in, 1 out]
  }
  n135 = call <vilib>:"Open Config Data.vi"("configuration file path"=w5) -> ("error out"=w9:errorcluster, "refnum"=w11:T16)  [unwired: 8 in, 1 out]
  n136 = property class="VI"(reference=w43) -> ("Name"=w42:string)  [unwired: 1 in, 2 out]
  n137 = property class="VI"(reference=w35) -> ("Name"=w28:string)  [unwired: 1 in, 2 out]
  n138 = Open VI Reference(type specifier VI Refnum (for type only)=refnum<vi> refnum, vi path=w42, options=128 ("选项")) -> (vi reference=w40:refnum<vi>, error out=w38:errorcluster)  [unwired: 3 in]
  n139 = call-poly <vilib>:"Read Key.vi"("section"="总磷总氮", "error in (no error)"=w9, "key"="总氮稀释倍数" ("section"), "refnum"=w11) -> ("error out"=w8:errorcluster, "value"=→"总氮稀释倍数":dbl, "refnum out"=w10:T16)  [unwired: 4 in, 1 out]
  n140 = call-by-ref "?"(reference=w40, error in=w38) -> (reference out=w36:refnum<vi>, error out=w37:errorcluster)  [unwired: 12 in]
  n141 = Open VI Reference(type specifier VI Refnum (for type only)=refnum<vi> refnum, vi path=w28, options=128 ("选项")) -> (vi reference=w30:refnum<vi>, error out=w32:errorcluster)  [unwired: 3 in]
  n142 = call "时间延迟2"() -> ("error out"=w12:errorcluster)  [unwired: 11 in]
  n143 = call-by-ref "?"(reference=w30, error in=w32) -> (reference out=w34:refnum<vi>, error out=w33:errorcluster)  [unwired: 12 in]
  n144 = Close Reference(reference=w36, error in (no error)=w37) -> ()  [unwired: 1 out]
  n145 = Close Reference(reference=w34, error in (no error)=w33) -> ()  [unwired: 1 out]
  n146 = call "总磷氨氮MB_api.vi"("STEP"=enum16{"open", "read", "write", "close"}."open", "Error in"=w12) -> ("error out"=w19:errorcluster)  [unwired: 7 in, 2 out]
  n147 = call <vilib>:"Close Config Data.vi"("error in (no error)"=w8, "refnum"=w10) -> ("error out"=w3:errorcluster)  [unwired: 8 in, 1 out]
  n148 = control-ref of="测量模式下拉列表"() -> (w24:refnum<vi>)
  n149 = control-ref of="量程切换阈值"() -> (w22:refnum<vi>)
  n150 = control-ref of="参数下拉列表"() -> (w25:refnum<vi>)
  n151 = control-ref of="量程下拉列表"() -> (w26:refnum<vi>)
  n152 = node-c288(w16) -> ()  [unwired: 1 out]
  n153 = control-ref of="备用系数"() -> (w21:refnum<vi>)
  n154 = control-ref of="公式"() -> (w23:refnum<vi>)
  n155 = Obtain Queue(name (unnamed)="TP" ("名称（未命名）"), element data type=cluster{"命令":string, "data":variant} {"命令"="", "data"=variant}) -> (queue out=w46:refnum<queue>, error out=w47:errorcluster)  [unwired: 3 in, 1 out]
  n156 = while {
    tunnel: w46 -> [w306]
    tunnel: w26 -> [w305]
    tunnel: w25 -> [w304]
    tunnel: w24 -> [w303]
    tunnel: w23 -> [w302]
    tunnel: w22 -> [w301]
    tunnel: w21 -> [w300]
    tunnel: w19 -> [_]
    tunnel: w3 -> [w299]
    stop <- FALSE stop-if-true
    n157 = event shown="[4] \"停止\": 值改变" {
      selector: _ -> [_ _ _ _ _ _ _ _ _ _ _ _ _ _ _ _]
      dyn-events: _ -> [_ _ _ _ _ _ _ _ _ _ _ _ _ _ _ _]
      timeout: _ -> [_ _ _ _ _ _ _ _ _ _ _ _ _ _ _ _]
      tunnel: w306 -> [_ w310 _ w321 w325 _ _ _ _ _ _ _ _ _ _ _]
      tunnel: w305 -> [_ _ _ _ _ _ _ _ _ w378 _ w398 w407 _ _ _]
      tunnel: w304 -> [_ _ _ _ _ _ _ _ _ w376 _ w396 w409 w417 w424 _]
      tunnel: w303 -> [_ _ _ _ _ _ _ _ _ w377 _ w397 w408 _ _ _]
      tunnel: w302 -> [_ _ _ _ _ _ _ _ _ w372 _ _ _ _ _ _]
      tunnel: w301 -> [_ _ _ _ _ _ _ _ _ _ _ w392 _ _ _ _]
      tunnel: w300 -> [_ _ _ _ _ _ _ _ _ _ _ _ _ w415 _ _]
      tunnel: w299 -> [_ _ _ _ _ _ _ _ _ _ _ _ _ _ _ _]
      event Timeout {
        n158 = event-data() -> ()  [unwired: 1 in, 3 out]
      }
      event "手动启动": Value Change {
        n159 = event-data() -> ()  [unwired: 1 in, 6 out]
        n160 = call "总磷氨氮启动参数对话框.vi"() -> ("确认"=w308:bool, "元素"=w309:cluster{"命令":string, "data":variant})  [unwired: 10 in]
        n161 = case shown="真" w308 {
          tunnel: w310 -> [_ w312]
          tunnel: w309 -> [_ w311]
          frame False {
          }
          frame True {
            n162 = Enqueue Element(queue=w312, element=w311) -> ()  [unwired: 2 in, 3 out]
          }
        }
      }
      event "定时启动": Mouse Down {
        n163 = event-data() -> ()  [unwired: 1 in, 6 out]
        n164 = call "定时启动对话框.vi"() -> ("设置值"=→"设置值":dbl, "确定输出"=→"定时启动":bool)  [unwired: 10 in]
      }
      event "单步测试": Value Change {
        w316 = u16 1 items=["总磷"=1, "氨氮"=3] ("站号")
        n165 = event-data() -> ()  [unwired: 1 in, 6 out]
        n166 = Bundle("站号"=w316, "总磷氨氮调试"="总磷氨氮调试") -> (w315:cluster{"站号":u16, "总磷氨氮调试":u16[]})  [unwired: 1 in]
        n167 = Bundle By Name(cluster=cluster{"命令":string, "data":variant} {"命令"="", "data"=variant} ("元素"), "命令"="debug", "data"=w315) -> (w318:cluster{"命令":string, "data":variant})
        n168 = Enqueue Element(queue=w321, element=w318) -> ()  [unwired: 2 in, 3 out]
      }
      event "停止": Value Change {
        n169 = event-data() -> ()  [unwired: 1 in, 6 out]
        n170 = Enqueue Element(queue=w325, element=cluster{"命令":string, "data":variant} {"命令"="启动", "data"=variant(cluster{"站号":u16, "控制命令输出":u16[]} {"站号"=1, "控制命令输出"=[2816]})} ("元素")) -> (queue out=w322:refnum<queue>)  [unwired: 2 in, 2 out]
        n171 = Enqueue Element(queue=w322, element=cluster{"命令":string, "data":variant} {"命令"="启动", "data"=variant(cluster{"站号":u16, "控制命令输出":u16[]} {"站号"=2, "控制命令输出"=[2816]})} ("元素")) -> ()  [unwired: 2 in, 3 out]
      }
      event "设置": Value Change {
        n172 = event-data() -> ()  [unwired: 1 in, 6 out]
        n173 = property on="窗格" class="Pane"("Origin"=T5 {"Horizontal"=0, "Vertical"=628} ("原点")) -> ()  [unwired: 2 in, 2 out]
      }
      event "返回": Value Change {
        n174 = event-data() -> ()  [unwired: 1 in, 6 out]
        n175 = property on="窗格" class="Pane"("Origin"=T5 {"Horizontal"=0, "Vertical"=0} ("原点")) -> ()  [unwired: 2 in, 2 out]
      }
      event "标液浓度1", "测量吸光度1", "测量吸光度2", "标液浓度2", "测量吸光度3", "标液浓度3", "测量吸光度4", "标液浓度4", "测量吸光度5", "标液浓度5", "样品1启用", "样品3启用", "样品4启用", "样品5启用", "样品2启用", "模型", "method", "样品1 F0", "样品1 F1", "样品2 F1", "样品2 F0", "样品3 F1", "样品4 F0", "样品4 F1", "样品5 F1", "样品5 F0", "精度": Value Change {
        n176 = event-data() -> ()  [unwired: 1 in, 6 out]
        n177 = formula code="E=log(F0/F1);"("F0"="样品1 F0", "F1"="样品1 F1") -> ("E"=w349:dbl)
        "测量吸光度1" <- w349
        n178 = formula code="E=log(F0/F1);"("F0"="样品2 F0", "F1"="样品2 F1") -> ("E"=w346:dbl)
        "测量吸光度2" <- w346
        n179 = formula code="E=log(F0/F1);"("F0"="样品3 F0", "F1"="样品3 F1") -> ("E"=w343:dbl)
        "测量吸光度3" <- w343
        n180 = formula code="E=log(F0/F1);"("F0"="样品4 F0", "F1"="样品4 F1") -> ("E"=w340:dbl)
        "测量吸光度4" <- w340
        n181 = formula code="E=log(F0/F1);"("F0"="样品5 F0", "F1"="样品5 F1") -> ("E"=w337:dbl)
        "测量吸光度5" <- w337
        n182 = Replace Array Subset(array=dbl[] [0.0, 0.0, 0.0, 0.0, 0.0] ("数组"), new element #1="标液浓度1", new element #2="标液浓度2", new element #3="标液浓度3", new element #4="标液浓度4", new element #5="标液浓度5") -> (w334:dbl[])  [unwired: 5 in]
        n183 = Replace Array Subset(array=dbl[] [0.0, 0.0, 0.0, 0.0, 0.0] ("数组"), new element #1=w349, new element #2=w346, new element #3=w343, new element #4=w340, new element #5=w337) -> (w333:dbl[])  [unwired: 5 in]
        n184 = Replace Array Subset(array=bool[] [FALSE, FALSE, FALSE, FALSE, FALSE] ("数组"), new element #1="样品1启用", new element #2="样品2启用", new element #3="样品3启用", new element #4="样品4启用", new element #5="样品5启用") -> (w332:bool[])  [unwired: 5 in]
        n185 = call "线性公式.vi"("精度"="精度", "模型"="模型", "method"="method", "启用"=w332, "监测浓度"=w333, "标液浓度"=w334) -> ("XY图"=→"XY图":cluster{"X Values":dbl[], "Y Values":dbl[]}[], "r^2"=→"r^2":dbl, "拟合方程"=→"拟合公式":string)  [unwired: 3 in]
      }
      event "标液浓度1", "标液浓度2", "标液浓度3", "标液浓度4", "标液浓度5", "样品1 F0", "样品1 F1", "样品2 F1", "样品2 F0", "样品3 F1", "样品3 F0", "样品4 F0", "样品4 F1", "样品5 F0", "样品5 F1", "精度", "公式.X^2", "公式.X", "公式.b", "量程切换阈值.阈值", "量程切换阈值.标液浓度", "备用系数.量程上限", "备用系数.量程下限", "备用系数.检出限", "备用系数.精度", "总氮稀释倍数": Mouse Down {
        n186 = event-data() -> ("CtlRef"=w368:refnum<vi>)  [unwired: 1 in, 5 out]
        n187 = property class="DigNum (严格)"(reference=w368) -> (reference out=w366:refnum<vi>, "Value"=w367:dbl)  [unwired: 1 in, 1 out]
        n188 = call "数字键盘.vi"("OldNumber"=w367) -> ("NewNumber"=w365:sgl)
        n189 = property class="DigNum (严格)"(reference=w366, "Val(Sgnl)"=w365) -> ()  [unwired: 1 in, 2 out]
      }
      event "读公式": Value Change {
        n190 = event-data() -> ()  [unwired: 1 in, 6 out]
        n191 = property class="Enum (严格)"(reference=w376) -> ("Value"=w375:enum16{"总磷", "总氮"})  [unwired: 1 in, 2 out]
        n192 = property class="Enum (严格)"(reference=w377) -> ("Value"=w374:enum16{"水样测量", "空白核查", "跨度核查", "标样核查", "加标回收"})  [unwired: 1 in, 2 out]
        n193 = property class="Enum (严格)"(reference=w378) -> ("Value"=w373:enum16{"低量程", "高量程"})  [unwired: 1 in, 2 out]
        n194 = call "总磷氨氮公式读取.vi"("量程"=w373, "测量模式"=w374, "测量参数"=w375) -> ("error out"=w370:errorcluster, "公式"=w371:cluster{"X^2":dbl, "X":dbl, "b":dbl})  [unwired: 7 in]
        n195 = property class="Clust (严格)"(reference=w372, "Value"=w371) -> ()  [unwired: 1 in, 2 out]
        n196 = case shown="错误" w370 {
          tunnel: ["读取成功" ("消息") "读取失败" ("消息")] -> w369
          frame No Error {
          }
          frame Error {
          }
        }
        n197 = One Button Dialog(message=w369) -> ()  [unwired: 1 in, 1 out]
      }
      event "写公式": Value Change {
        n198 = event-data() -> ()  [unwired: 1 in, 6 out]
        n199 = call "总磷氨氮公式写入.vi"("公式"="公式", "量程"="量程下拉列表", "测量模式"="测量模式下拉列表", "测量参数"="参数下拉列表") -> ("error out"=w383:errorcluster)  [unwired: 7 in]
        n200 = case shown="无错误" w383 {
          tunnel: ["写入成功" ("消息") "写入失败" ("消息")] -> w384
          frame No Error {
          }
          frame Error {
          }
        }
        n201 = One Button Dialog(message=w384) -> ()  [unwired: 1 in, 1 out]
      }
      event "量程切换阈值读取": Value Change {
        n202 = event-data() -> ()  [unwired: 1 in, 6 out]
        n203 = property class="Enum (严格)"(reference=w396) -> ("Value"=w395:enum16{"总磷", "总氮"})  [unwired: 1 in, 2 out]
        n204 = property class="Enum (严格)"(reference=w397) -> ("Value"=w394:enum16{"水样测量", "空白核查", "跨度核查", "标样核查", "加标回收"})  [unwired: 1 in, 2 out]
        n205 = property class="Enum (严格)"(reference=w398) -> ("Value"=w393:enum16{"低量程", "高量程"})  [unwired: 1 in, 2 out]
        n206 = call "总磷氨氮量程读取.vi"("量程"=w393, "测量模式"=w394, "测量参数"=w395) -> ("error out"=w389:errorcluster, "量程切换阈值"=w391:cluster{"阈值":dbl, "标液浓度":dbl})  [unwired: 7 in]
        n207 = property class="Clust (严格)"(reference=w392, "Value"=w391) -> ()  [unwired: 1 in, 2 out]
        n208 = case shown="错误" w389 {
          tunnel: ["读取成功" ("消息") "读取失败" ("消息")] -> w390
          frame No Error {
          }
          frame Error {
          }
        }
        n209 = One Button Dialog(message=w390) -> ()  [unwired: 1 in, 1 out]
      }
      event "量程切换阈值写入": Value Change {
        n210 = event-data() -> ()  [unwired: 1 in, 6 out]
        n211 = property class="Enum (严格)"(reference=w409) -> ("Value"=w406:enum16{"总磷", "总氮"})  [unwired: 1 in, 2 out]
        n212 = property class="Enum (严格)"(reference=w408) -> ("Value"=w405:enum16{"水样测量", "空白核查", "跨度核查", "标样核查", "加标回收"})  [unwired: 1 in, 2 out]
        n213 = property class="Enum (严格)"(reference=w407) -> ("Value"=w404:enum16{"低量程", "高量程"})  [unwired: 1 in, 2 out]
        n214 = call "总磷氨氮量程写入.vi"("量程切换阈值"="量程切换阈值", "量程"=w404, "测量模式"=w405, "测量参数"=w406) -> ("error out"=w401:errorcluster)  [unwired: 7 in]
        n215 = case shown="无错误" w401 {
          tunnel: ["写入成功" ("消息") "写入失败" ("消息")] -> w402
          frame No Error {
          }
          frame Error {
          }
        }
        n216 = One Button Dialog(message=w402) -> ()  [unwired: 1 in, 1 out]
      }
      event "备用系数读取": Value Change {
        n217 = event-data() -> ()  [unwired: 1 in, 6 out]
        n218 = property class="Enum (严格)"(reference=w417) -> ("Value"=w416:enum16{"总磷", "总氮"})  [unwired: 1 in, 2 out]
        n219 = call "总磷氨氮备用系数读取.vi"("测量参数"=w416) -> ("error out"=w412:errorcluster, "备用系数"=w414:T1)  [unwired: 9 in]
        n220 = property class="Clust (严格)"(reference=w415, "Value"=w414) -> ()  [unwired: 1 in, 2 out]
        n221 = case shown="错误" w412 {
          tunnel: ["读取成功" ("消息") "读取失败" ("消息")] -> w413
          frame No Error {
          }
          frame Error {
          }
        }
        n222 = One Button Dialog(message=w413) -> ()  [unwired: 1 in, 1 out]
      }
      event "备用系数写入": Value Change {
        n223 = event-data() -> ()  [unwired: 1 in, 6 out]
        n224 = property class="Enum (严格)"(reference=w424) -> ("Value"=w423:enum16{"总磷", "总氮"})  [unwired: 1 in, 2 out]
        n225 = call "总磷氨氮备用系数写入.vi"("备用系数"="备用系数", "测量参数"=w423) -> ("error out"=w420:errorcluster)  [unwired: 9 in]
        n226 = case shown="无错误" w420 {
          tunnel: ["写入成功" ("消息") "写入失败" ("消息")] -> w421
          frame No Error {
          }
          frame Error {
          }
        }
        n227 = One Button Dialog(message=w421) -> ()  [unwired: 1 in, 1 out]
      }
      event "总氮稀释倍数": Value Change {
        n228 = event-data() -> ()  [unwired: 1 in, 6 out]
        n229 = call <vilib>:"Application Directory.vi"() -> ("Application Directory"=w434:path)
        n230 = Build Path(base path=w434, name or relative path="data\\Set.ini" ("名称或相对路径")) -> (appended path=w436:path)
        n231 = local read "总氮稀释倍数"() -> (w429:dbl)
        n232 = call <vilib>:"Open Config Data.vi"("configuration file path"=w436) -> ("error out"=w431:errorcluster, "refnum"=w433:T16)  [unwired: 8 in, 1 out]
        n233 = global write "VAR总磷氨氮全局变量.vi" "总氮稀释倍数"(w429) -> ()
        n234 = call-poly <vilib>:"Write Key.vi"("section"="总磷总氮", "error in (no error)"=w431, "value"=w429, "key"="总氮稀释倍数" ("section"), "refnum"=w433) -> ("error out"=w430:errorcluster, "refnum out"=w432:T16)  [unwired: 4 in, 1 out]
        n235 = call <vilib>:"Close Config Data.vi"("error in (no error)"=w430, "refnum"=w432) -> ()  [unwired: 8 in, 2 out]
      }
    }
  }
  n236 = while {
    tunnel: w46 -> [w453]
    tunnel: w47 -> [_]
    shift-right: [w445] -> _
    shift-left: enum16{"总磷", "总氮"}."总磷" ("枚举") -> [w447]
    stop <- FALSE stop-if-true
    # "试剂填充 172 \n管路清洗108\n氨氮92\n总磷131\n总磷海水147\n总氮76\n总氮海水92"
    n237 = case shown="\"总氮\", 默认" w447 {
      selector: w447 -> [w462 w464]
      tunnel: [w463 w465] -> w448
      tunnel: [w462 w464] -> w446
      frame "总氮", Default {
        w463 = u16 2 items=["总磷"=1, "总氮"=2] ("站号")
      }
      frame "总磷" {
        w465 = u16 1 items=["总磷"=1, "氨氮"=3] ("站号")
      }
    }
    n238 = Wait (ms)(milliseconds to wait=u32 1000 ("等待时间（毫秒）")) -> ()  [unwired: 1 out]
    n239 = Bundle By Name(cluster=cluster{"命令":string, "data":variant} {"命令"="", "data"=variant} ("元素"), "命令"="读状态告警区", "data"=w448) -> (w455:cluster{"命令":string, "data":variant})
    n240 = global read "VAR总磷氨氮全局变量.vi" "状态告警区"() -> (w437:T3)
    n241 = Unbundle By Name(w437) -> ("系统时间"=w444:timestamp)
    n242 = Enqueue Element(queue=w453, element=w455) -> (queue out=w449:refnum<queue>)  [unwired: 2 in, 2 out]
    n243 = Get Date/Time In Seconds() -> (seconds since 1Jan1904=w443:timestamp)
    n244 = Subtract(x=w443, y=w444) -> (x-y=w442:dbl)
    n245 = Bundle By Name(cluster=cluster{"命令":string, "data":variant} {"命令"="", "data"=variant} ("元素"), "命令"="读测量数据区", "data"=w448) -> (w451:cluster{"命令":string, "data":variant})
    n246 = Absolute Value(x=w442) -> (abs(x)=w441:dbl)
    n247 = Enqueue Element(queue=w449, element=w451) -> (queue out=w438:refnum<queue>)  [unwired: 2 in, 2 out]
    n248 = Greater Or Equal?(x=w441, y=120.0) -> (x >= y?=w439:bool)
    n249 = Increment(x=w446) -> (x+1=w445:enum16{"总磷", "总氮"})
    n250 = case shown="真" w439 {
      tunnel: w438 -> [_ w460]
      frame False {
      }
      frame True {
        n251 = call "总磷氨氮启动命令.vi"("参数"=T17 {"站号"=3, "量程切换"=enum."AUTO", "控制命令"=enum."校时", "模式设置"=enum."待机", "测量间隔"=0}) -> ("启动命令"=w459:cluster{"命令":string, "data":variant})  [unwired: 10 in]
        n252 = Enqueue Element(queue=w460, element=w459) -> ()  [unwired: 2 in, 3 out]
      }
    }
  }
  n253 = while {
    tunnel: w46 -> [w469]
    shift-right: [w470] -> _
    shift-left: T4."待机" -> [w471]
    shift-right: [w467] -> _
    shift-left: u32 0 ("等待时间（毫秒）") -> [w468]
    stop <- FALSE stop-if-true
    n254 = Wait (ms)(milliseconds to wait=u32 1000 ("等待时间（毫秒）")) -> ()  [unwired: 1 out]
    n255 = local read "定时启动"() -> (w472:bool)
    n256 = case shown="真" w472 {
      tunnel: w471 -> [_ w481]
      tunnel: [T4."待机" w480] -> w470
      tunnel: w469 -> [_ w479]
      tunnel: w468 -> [_ w478]
      tunnel: [_ w477] -> w467
      tunnel: [_ w476] -> w466
      frame False {
      }
      frame True {
        n257 = case shown="\"启动总磷\"" w481 {
          tunnel: [T4."启动氨氮" w488 w494 w508 w515 w534] -> w480
          tunnel: w479 -> [_ w493 _ w514 _ _]
          tunnel: w478 -> [_ _ _ _ _ w536]
          tunnel: [_ _ _ _ _ w528] -> w477
          tunnel: ["待机" ("字符串") "启动总氮" ("字符串") "总氮运行中" ("字符串") "启动总磷" ("字符串") "总磷运行中" ("字符串") w526] -> w476
          frame "待机", Default {
          }
          frame "启动氨氮" {
            n258 = call "总磷氨氮启动命令.vi"("参数"=T18 {"站号"=2, "量程切换"=enum."AUTO", "控制命令"=enum."启动测量", "模式设置"=enum."待机", "测量间隔"=0}) -> ("启动命令"=w486:cluster{"命令":string, "data":variant})  [unwired: 10 in]
            n259 = Enqueue Element(queue=w493, element=w486) -> ()  [unwired: 2 in, 3 out]
            n260 = global read "VAR总磷氨氮全局变量.vi" "状态告警区"() -> (w492:T3)
            n261 = Unbundle By Name(w492) -> ("工作状态"=w491:T7)
            n262 = Not Equal To 0?(x=w491) -> (x != 0?=w490:bool)
            n263 = Select(t=T4."氨氮测量中", s=w490, f=T4."启动氨氮") -> (s? t:f=w488:T4)
          }
          frame "氨氮测量中" {
            n264 = global read "VAR总磷氨氮全局变量.vi" "状态告警区"() -> (w497:T3)
            n265 = Unbundle By Name(w497) -> ("工作状态"=w495:T7, "id"=w496:u16)
            n266 = case shown="默认" w495 {
              tunnel: w496 -> [_ w502]
              tunnel: [T4."启动总磷" w501] -> w494
              frame "空闲" {
                n267 = Wait (ms)(milliseconds to wait=u32 8000 ("等待时间（毫秒）")) -> ()  [unwired: 1 out]
              }
              frame Default {
                n268 = case shown="76, 默认" w502 {
                  tunnel: [T4."氨氮测量中" T4."总磷测量中"] -> w501
                  frame 76, Default {
                  }
                  frame 131 {
                  }
                }
              }
            }
          }
          frame "启动总磷" {
            n269 = call "总磷氨氮启动命令.vi"("参数"=T18 {"站号"=1, "量程切换"=enum."AUTO", "控制命令"=enum."启动测量", "模式设置"=enum."待机", "测量间隔"=0}) -> ("启动命令"=w507:cluster{"命令":string, "data":variant})  [unwired: 10 in]
            n270 = Enqueue Element(queue=w514, element=w507) -> ()  [unwired: 2 in, 3 out]
            n271 = global read "VAR总磷氨氮全局变量.vi" "状态告警区"() -> (w509:T3)
            n272 = Unbundle By Name(w509) -> ("工作状态"=w510:T7)
            n273 = Not Equal To 0?(x=w510) -> (x != 0?=w511:bool)
            n274 = Select(t=T4."总磷测量中", s=w511, f=T4."启动总磷") -> (s? t:f=w508:T4)
          }
          frame "总磷测量中" {
            n275 = global read "VAR总磷氨氮全局变量.vi" "状态告警区"() -> (w518:T3)
            n276 = Unbundle By Name(w518) -> ("工作状态"=w516:T7, "id"=w517:u16)
            n277 = case shown="默认" w516 {
              tunnel: w517 -> [_ w523]
              tunnel: [T4."延时" w522] -> w515
              frame "空闲" {
                n278 = Wait (ms)(milliseconds to wait=u32 8000 ("等待时间（毫秒）")) -> ()  [unwired: 1 out]
              }
              frame Default {
                n279 = case shown="76, 默认" w523 {
                  tunnel: [T4."氨氮测量中" T4."总磷测量中"] -> w522
                  frame 76, Default {
                  }
                  frame 131 {
                  }
                }
              }
            }
          }
          frame "延时" {
            n280 = local read "设置值"() -> (w531:dbl)
            n281 = Increment(x=w536) -> (x+1=w528:u32)
            n282 = Add(x=w531, y=10.0) -> (x+y=w529:dbl)
            n283 = Greater Or Equal?(x=w528, y=w529) -> (x >= y?=w535:bool)
            n284 = Select(t=T4."待机", s=w535, f=T4."延时") -> (s? t:f=w534:T4)
            n285 = Format Into String(format string="延时计时中%d秒" ("格式字符串"), w528) -> (resulting string=w526:string)  [unwired: 2 in, 1 out]
          }
        }
      }
    }
    "字符串" <- w466
  }
